vi "Write Length.vi"(8 "error in (no error)":errorcluster, 10 "Length":u64, 11 "Abstruct Data Type in":refnum<class "Abstruct Data Type.lvclass">) -> (0 "error out":errorcluster, 3 "Abstruct Data Type out":refnum<class "Abstruct Data Type.lvclass">)   [LabVIEW 2020, in "Abstruct Data Type.lvclass"]
uses:
  Abstruct Data Type.lvclass
  Abstruct Data Type.lvclass/Abstruct Data Type.ctl
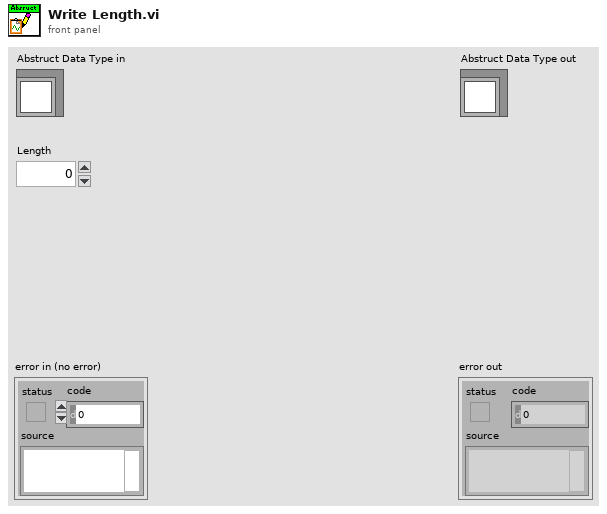
[diagram p1: front panel]
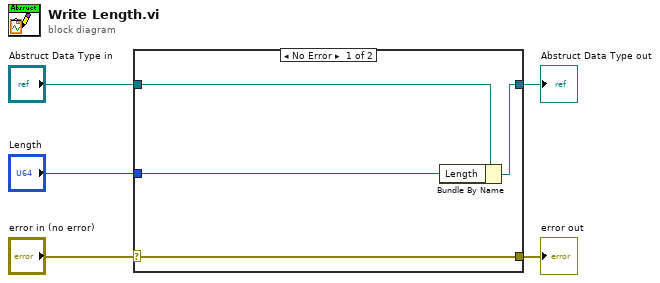
[diagram p0: block diagram]
diagram:
  n1 = case shown="No Error" "error in (no error)" {
    selector: "error in (no error)" -> [w9 w10]
    tunnel: [w9 w10] -> w4
    tunnel: [w7 w11] -> w2
    tunnel: "Abstruct Data Type in" -> [w8 w11]
    tunnel: "Length" -> [w6 _]
    frame No Error {
      n2 = Bundle By Name(cluster=w8, "Length"=w6) -> (w7:refnum<class "Abstruct Data Type.lvclass">)
    }
    frame Error {
    }
  }
  "error out" <- w4
  "Abstruct Data Type out" <- w2
